vi "WaitIfNeeded.vi"(6 "retry":bool, 8 "stopping":bool, 10 "wait":refnum<k4>, 11 "_timeout (ms) in":i32) -> (0 "stop loop":bool, 2 "timed out":bool, 3 "_timeout (ms) out":i32)   [LabVIEW 2019, in "_ChannelSupport.lvlib"]
uses:
  _ChannelSupport.lvlib
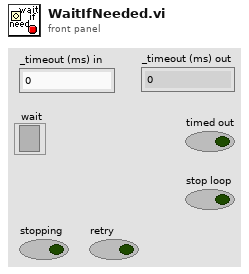
[diagram p1: front panel]
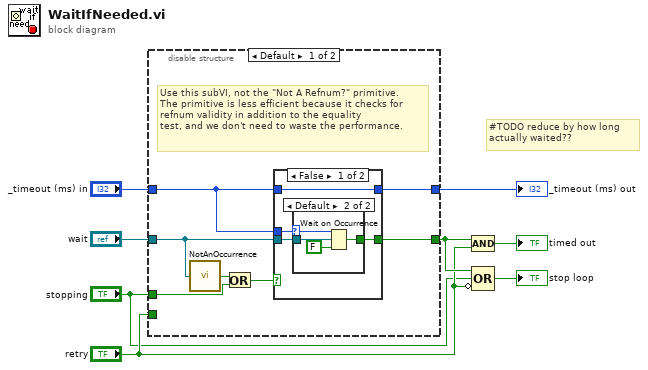
[diagram p0: block diagram]
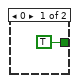
[diagram p2: hidden frame]
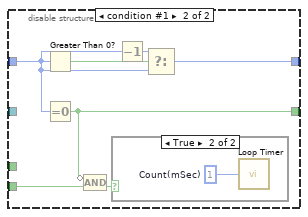
[diagram p4: hidden frame]
diagram:
  # "#TODO reduce by how long\nactually waited??"
  n1 = disable-structure shown="Default" {
    disable-tunnel: "wait" -> [w10 _]
    disable-tunnel: "_timeout (ms) in" -> [w11 w31]
    disable-tunnel: [w15 w28] -> w4
    disable-tunnel: "retry" -> [_ w27]
    disable-tunnel: [w12 w30] -> w8
    disable-tunnel: "stopping" -> [w13 _]
    frame condition #0 (active) {
      # "Use this subVI, not the \"Not A Refnum?\" primitive.\nThe primitive is less efficient because it checks for refnum validity in addition to the equality\ntest, and we don't need to waste the performance."
      n2 = call "NotAnOccurrence.vi"("occurrence refnum"=w10) -> ("not an occurrence?"=w9:bool)
      n3 = Or(x=w9, y=w13) -> (x .or. y?=w14:bool)
      n4 = case shown="False" w14 {
        tunnel: w10 -> [w19 _]
        tunnel: w11 -> [w18 _]
        tunnel: [w17 _] -> w15
        tunnel: [w16 w25] -> w12
        tunnel: w11 -> [w16 w25]
        frame False {
          n5 = case shown="Default" w18 {
            selector: w18 -> [_ w23]
            tunnel: w19 -> [_ w24]
            tunnel: [TRUE ("timed out") w21] -> w17
            frame 0 {
            }
            frame Default {
              n6 = Wait on Occurrence(1:FALSE ("ignore previous (T)"), 2:w24, 3:w23) -> (0:w21:bool)
            }
          }
        }
        frame True {
        }
      }
    }
    frame condition #1 {
      n7 = Greater Than 0?(x=w31) -> (x > 0?=w29:bool)
      n8 = Equal To 0?(x=w31) -> (x = 0?=w28:bool)
      n9 = Compound Arithmetic op=AND(invert w28, w27) -> (w26:bool)
      n10 = case shown="True" w26 {
        frame False {
        }
        frame True {
          w33 = u32 1  # Count(mSec)
          n11 = call "Loop Timer"("Count(mSec)"=w33) -> ()  [unwired: 1 out]
        }
      }
      n12 = Decrement(x=w31) -> (x-1=w32:i32)
      n13 = Select(t=w32, s=w29, f=w31) -> (s? t:f=w30:i32)
    }
  }
  "_timeout (ms) out" <- w8
  n14 = Compound Arithmetic op=AND(w4, "retry") -> (→"timed out":bool)
  n15 = Compound Arithmetic op=OR(w4, "stopping", invert "retry") -> (→"stop loop":bool)
